vi "ActiveObjects_DynamicEvents_ControlWindow_5x6x5_Singleton.vi"(5 "ShowProcessWindow":bool, 11 "Error In":errorcluster) -> (15 "Error Out":errorcluster)   [LabVIEW 2020]
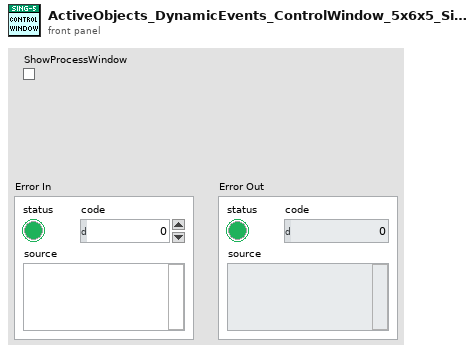
[diagram p1: front panel]
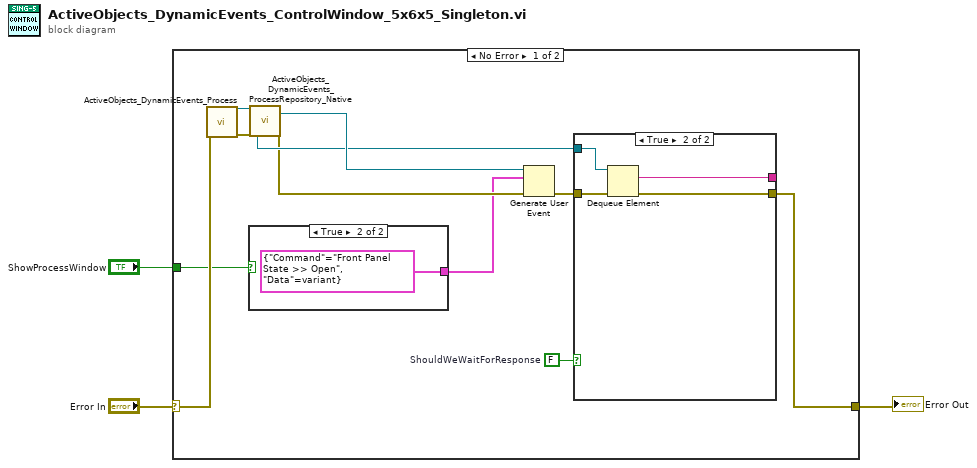
[diagram p0: block diagram]
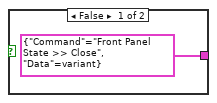
[diagram p2: hidden frame]
diagram:
  n1 = case shown="No Error" "Error In" {
    selector: "Error In" -> [w7 w22]
    tunnel: [w9 w22] -> w2
    tunnel: "ShowProcessWindow" -> [w5 _]
    frame No Error {
      w13 = FALSE  # ShouldWeWaitForResponse
      n2 = call <resource>:"ActiveObjects_DynamicEvents_Process.vi"("error in"=w7) -> ("reference out"=w8:refnum<class>, "error out"=w6:errorcluster)  [unwired: 17 in]
      n3 = case shown="True" w5 {
        tunnel: [cluster{"Command":string, "Data":variant} {"Command"="Front Panel State >> Close", "Data"=variant} ("MessageToProcess") cluster{"Command":string, "Data":variant} {"Command"="Front Panel State >> Open", "Data"=variant} ("MessageToProcess")] -> w4
        frame False {
        }
        frame True {
        }
      }
      n4 = call <resource>:"ActiveObjects_DynamicEvents_ProcessRepository_Native.vi"("reference in"=w8, "Error In"=w6) -> ("QueueFromProcess"=w11:refnum<queue>, "EventsToProcess"=w14:refnum<user-event>, "Error Out"=w10:errorcluster)  [unwired: 10 in, 5 out]
      n5 = Generate User Event(user event=w14, event data cluster=w4, error in=w10) -> (error out=w12:errorcluster)  [unwired: 1 in, 1 out]
      n6 = case shown="True" w13 {
        tunnel: w12 -> [w17 w21]
        tunnel: w11 -> [_ w20]
        tunnel: [_ w19] -> _
        tunnel: [w17 w18] -> w9
        frame False {
        }
        frame True {
          n7 = Dequeue Element(queue=w20, error in (no error)=w21) -> (element=w19:string, error out=w18:errorcluster)  [unwired: 1 in, 2 out]
        }
      }
    }
    frame Error {
    }
  }
  "Error Out" <- w2
